vi "Serial Test.vi"() -> ()   [LabVIEW 2011]
uses:
  PID/Engine RPM/Engine RPM.lvclass
  PID/Throttle Position/Throttle Position.lvclass
  PID/Fuel Level Input/Fuel Level Input Folder/Fuel Level Input.lvclass
  PID/PID.lvclass
  PID/VIN/VIN Folder/VIN.lvclass
  <vilib>/Instr/_visa.llb/VISA Configure Serial Port (Instr).vi
panel:
  out "Fuel Level":dbl(knob) scale=0.0..100.0
  in  "Get All":bool
  out "Response":string
  out "Throttle":dbl(knob) scale=0.0..100.0
  out "Waveform Chart 2":cluster{"Result":dbl, "Result":dbl}(graph)
  out "RPM":dbl(knob) scale=0.0..5000.0
  out "Discard?":bool
  in  "milliseconds to wait":u32=250
  in  "VIN":bool
  in  "Polling":bool
  in  "Check All":bool
  out "number":u32
  in  "29-Bit CAN":bool[](array[boolean])
  in  "Send Button":bool
  in  "Command":string
  in  "Multicolumn Listbox 2":i32(listbox)=-1
  out "String":string="0100\r\r41 00 BE 7F A8 13 \r0120\r\r41 20 80 07 B0 11 \r0140\r\r41 40 FE D0 0C 00 \r0100\r41 00 BE 7F A8 13 \r0102\rNO DATA\r0103\r41 03 02 00 \r0104\r41 04 30 \r0105\r41 05 80 \r0106\r41 06 86 \r0109\rNO DATA\r010A\r41 0A 7D \r010B\r41 0B 22 \r010C\r41 0C 0A 1F \r010D\r41 0D 00 \r010E\r41 0E 8A \r010F\r41 0F 3D \r0110\r41 10 01 45 \r0112\rNO DATA\r0114\rNO DATA\r011B\rNO DATA\r011E\rNO DATA\r011F\r41 1F 03 A4 \r0120\r41 20 80 07 B0 11 \r012D\rNO DATA\r012E\r41 2E FF \r012F\r41 2F ED \r0130\r41 30 FF \r0132\rNO DATA\r0133\r41 33 65 \r013B\rNO DATA\r013F\rNO DATA\r0140\r41 40 FE D0 0C 00 \r0141\r41 41 00 07 E5 A5 \r0142\r41 42 37 FF \r0143\r41 43 00 29 \r0144\r41 44 7C AC \r0145\r41 45 04 \r0146\r41 46 31 \r0148\rNO DATA\r0149\r41 49 12 \r014B\rNO DATA\r0154\rNO DATA\r0155\r41 55 82 \r010C\r41 0C 0A 30 \r0111\r41 11 21 \r010C\r41 0C 0A 37 \r0111\r41 11 21 \r010C\r41 0C 0A 44 \r0111\r41 11 21 \r010C\r41 0C 0A 28 \r0111\r41 11 21 \r010C\r41 0C 0A 1B \r0111\r41 11 21 \r010C\r41 0C 0A 26 \r0111\r41 11 21 \r010C\r41 0C 0A 10 \r0111\r41 11 21 \r010C\r41 0C 0A 1B \r0111\r41 11 21 \r010C\r41 0C 0A 26 \r0111\r41 11 21 \r010C\r41 0C 0A 4F \r0111\r41 11 21 \r010C\r41 0C 0A 49 \r0111\r41 11 21 \r010C\r41 0C 0A 40 \r0111\r41 11 21 \r010C\r41 0C 0A 40 \r0111\r41 11 21 \r010C\r41 0C 0A 19 \r0111\r41 11 21 \r010C\r41 0C 0A 27 \r0111\r41 11 21 \r010C\r41 0C 0A 13 \r0111\r41 11 21 \r010C\r41 0C 09 FF \r0111\r41 11 21 \r010C\r41 0C 0A 20 \r0111\r41 11 21 \r010C\r41 0C 0A 50 \r0111\r41 11 21 \r010C\r41 0C 0A 38 \r0111\r41 11 21 \r010C\r41 0C 0A 18 \r0111\r41 11 21 \r010C\r41 0C 0A 0D \r0111\r41 11 21 \r010C\r41 0C 0A 26 \r0111\r41 11 21 \r010C\r41 0C 0A 30 \r0111\r41 11 21 \r010C\r41 0C 0A 29 \r0111\r41 11 21 \r010C\r41 0C 0A 31 \r0111\r41 11 21 \r010C\r41 0C 0A 24 \r0111\r41 11 21 \r010C\r41 0C 0A 26 \r0111\r41 11 21 \r010C\r41 0C 0A 23 \r0111\r41 11 21 \r010C\r41 0C 0A 25 \r0111\r41 11 21 \r010C\r41 0C 0A 14 \r0111\r41 11 21 \r010C\r41 0C 0A 39 \r0111\r41 11 21 \r010C\r41 0C 0A 0D \r0111\r41 11 21 \r010C\r41 0C 0A 00 \r0111\r41 11 21 \r010C\r41 0C 0A 29 \r0111\r41 11 21 \r010C\r41 0C 0A 25 \r0111\r41 11 21 \r010C\r41 0C 0A 22 \r0111\r41 11 21 \r010C\r41 0C 0A 2D \r0111\r41 11 21 \r010C\r41 0C 0A 40 \r0111\r41 11 21 \r010C\r41 0C 0A 44 \r0111\r41 11 21 \r010C\r41 0C 0A 30 \r0111\r41 11 21 \r010C\r41 0C 0A 2D \r0111\r41 11 21 \r010C\r41 0C 0A 33 \r0111\r41 11 21 \r010C\r41 0C 0A 17 \r0111\r41 11 21 \r010C\r41 0C 0A 34 \r0111\r41 11 21 \r010C\r41 0C 0A 2B \r0111\r41 11 21 \r010C\r41 0C 0A 46 \r0111\r41 11 21 \r010C\r41 0C 0A 1C \r0111\r41 11 21 \r010C\r41 0C 0A 10 \r0111\r41 11 21 \r010C\r41 0C 0A 2F \r0111\r41 11 21 \r010C\r41 0C 09 FB \r0111\r41 11 21 \r010C\r41 0C 0A 1B \r0111\r41 11 21 \r010C\r41 0C 0A 27 \r0111\r41 11 21 \r010C\r41 0C 0A 32 \r0111\r41 11 21 \r010C\r41 0C 0A 3D \r0111\r41 11 21 \r010C\r41 0C 0A 35 \r0111\r41 11 21 \r010C\r41 0C 0A 2E \r0111\r41 11 21 \r010C\r41 0C 0A 34 \r0111\r41 11 21 \r010C\r41 0C 0A 1E \r0111\r41 11 21 \r010C\r41 0C 0A 05 \r0111\r41 11 21 \r010C\r41 0C 0A 16 \r0111\r41 11 21 \r010C\r41 0C 0A 3B \r0111\r41 11 21 \r010C\r41 0C 0A 38 \r0111\r41 11 21 \r010C\r41 0C 0A 46 \r0111\r41 11 21 \r010C\r41 0C 0A 29 \r0111\r41 11 21 \r010C\r41 0C 0A 2F \r0111\r41 11 21 \r010C\r41 0C 0A 2C \r0111\r41 11 21 \r010C\r41 0C 0A 1D \r0111\r41 11 21 \r010C\r41 0C 0A 01 \r0111\r41 11 21 \r010C\r41 0C 0A 19 \r0111\r41 11 21 \r010C\r41 0C 0A 18 \r0111\r41 11 21 \r010C\r41 0C 0A 0F \r0111\r41 11 21 \r010C\r41 0C 0A 32 \r0111\r41 11 21 \r010C\r41 0C 0A 49 \r0111\r41 11 21 \r010C\r41 0C 0A 49 \r0111\r41 11 21 \r010C\r41 0C 0A 5A \r0111\r41 11 21 \r010C\r41 0C 0A 4F \r0111\r41 11 21 \r010C\r41 0C 0A 3C \r0111\r41 11 21 \r010C\r41 0C 0A 2A \r0111\r41 11 21 \r010C\r41 0C 0A 28 \r0111\r41 11 21 \r010C\r41 0C 0A 04 \r0111\r41 11 21 \r010C\r41 0C 0A 1B \r0111\r41 11 21 \r010C\r41 0C 0A 24 \r0111\r41 11 21 \r010C\r41 0C 0A 4B \r0111\r41 11 21 \r010C\r41 0C 0A 30 \r0111\r41 11 21 \r010C\r41 0C 0A 11 \r0111\r41 11 21 \r010C\r41 0C 0A 05 \r0111\r41 11 21 \r010C\r41 0C 0A 0C \r0111\r41 11 21 \r010C\r41 0C 0A 1E \r0111\r41 11 21 \r010C\r41 0C 0A 26 \r0111\r41 11 21 \r010C\r41 0C 0A 30 \r0111\r41 11 21 \r010C\r41 0C 0A 41 \r0111\r41 11 21 \r010C\r41 0C 0A 2C \r0111\r41 11 21 \r010C\r41 0C 0A 3B \r0111\r41 11 21 \r010C\r41 0C 0A 2F \r0111\r41 11 21 \r010C\r41 0C 0A 34 \r0111\r41 11 21 \r010C\r41 0C 0A 48 \r0111\r41 11 21 \r010C\r41 0C 0A 2B \r0111\r41 11 21 \r010C\r41 0C 0A 27 \r0111\r41 11 21 \r010C\r41 0C 0A 25 \r0111\r41 11 21 \r010C\r41 0C 0A 19 \r0111\r41 11 21 \r010C\r41 0C 0A 2C \r0111\r41 11 21 \r010C\r41 0C 0A 30 \r0111\r41 11 21 \r010C\r41 0C 0A 11 \r0111\r41 11 21 \r010C\r41 0C 0A 38 \r0111\r41 11 21 \r010C\r41 0C 0A 20 \r0111\r41 11 21 \r010C\r41 0C 0A 25 \r0111\r41 11 21 \r010C\r41 0C 0A 1C \r0111\r41 11 21 \r010C\r41 0C 0A 2B \r0111\r41 11 21 \r010C\r41 0C 0A 2E \r0111\r41 11 21 \r010C\r41 0C 0A 40 \r0111\r41 11 21 \r010C\r41 0C 0A 1A \r0111\r41 11 21 \r010C\r41 0C 0A 1F \r0111\r41 11 21 \r010C\r41 0C 0A 2F \r0111\r41 11 21 \r010C\r41 0C 0A 22 \r0111\r41 11 21 \r010C\r41 0C 0A 3C \r0111\r41 11 21 \r010C\r41 0C 0A 27 \r0111\r41 11 21 \r010C\r41 0C 0A 27 \r0111\r41 11 21 \r010C\r41 0C 0A 12 \r0111\r41 11 21 \r010C\r41 0C 0A 37 \r0111\r41 11 21 \r010C\r41 0C 0A 1E \r0111\r41 11 21 \r010C\r41 0C 0A 13 \r0111\r41 11 21 \r010C\r41 0C 0A 1C \r0111\r41 11 22 \r010C\r41 0C 0A 16 \r0111\r41 11 22 \r010C\r41 0C 0A 00 \r0111\r41 11 22 \r010C\r41 0C 0A 1B \r0111\r41 11 22 \r0902\r\r014 \r0902\r\r014 \r0902\r\r014 \r0902\r\r014 \r0900\r\r49 00 55 40 00 00 \r0901\r\rNO DATA\r0902\r\r014 \r"
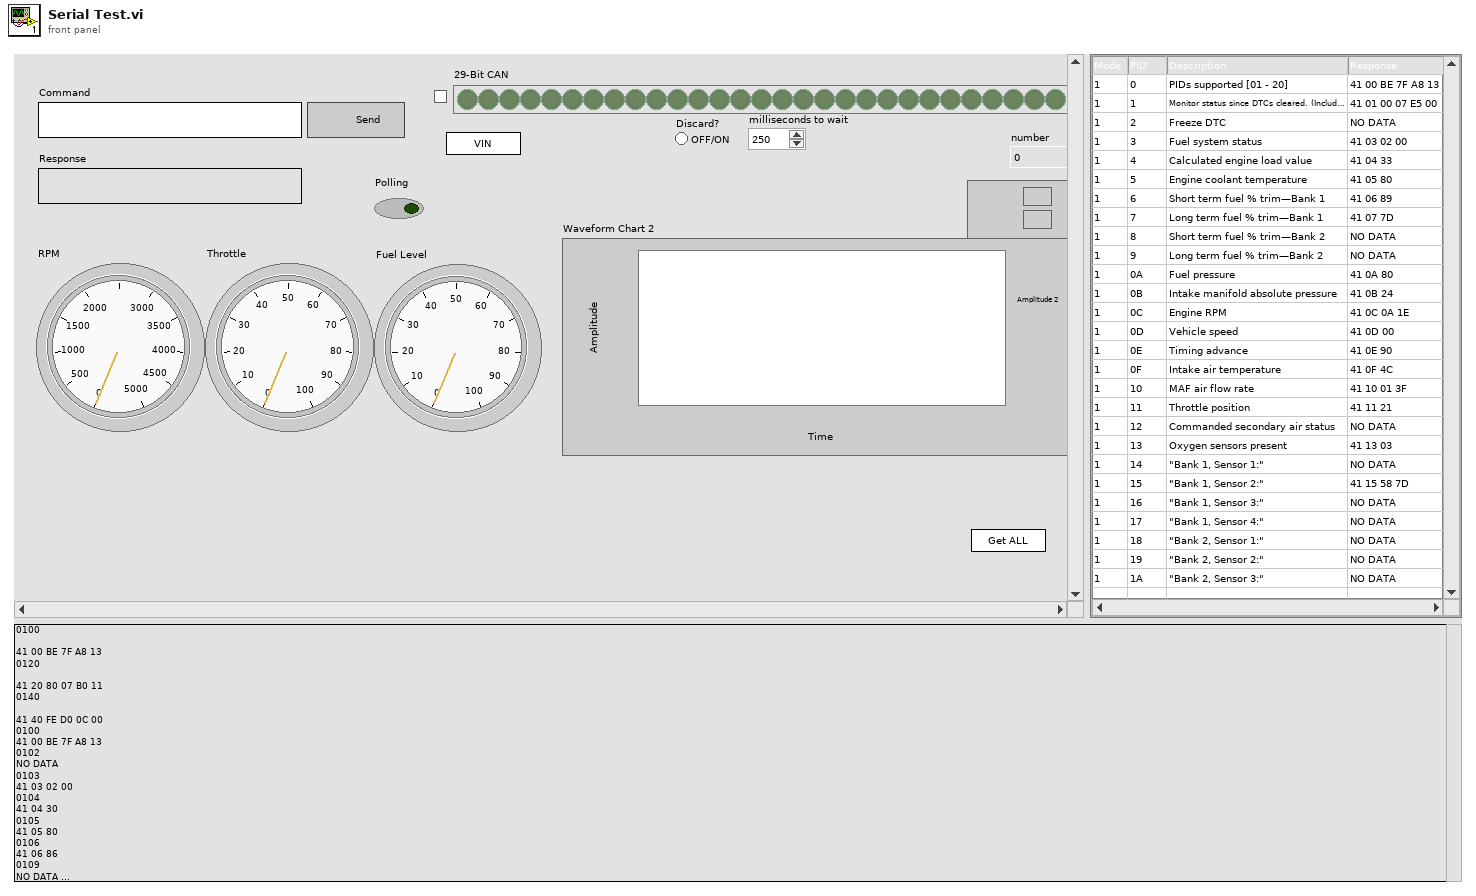
[diagram p1: front panel]
types:
  T1 = typedef "LVPoint32TypeDef.ctl" = cluster{"Horizontal":i32, "Vertical":i32}
  T2 = typedef "LVRowAndColumnTypeDef.ctl" = cluster{"Row":i32, "Column":i32}
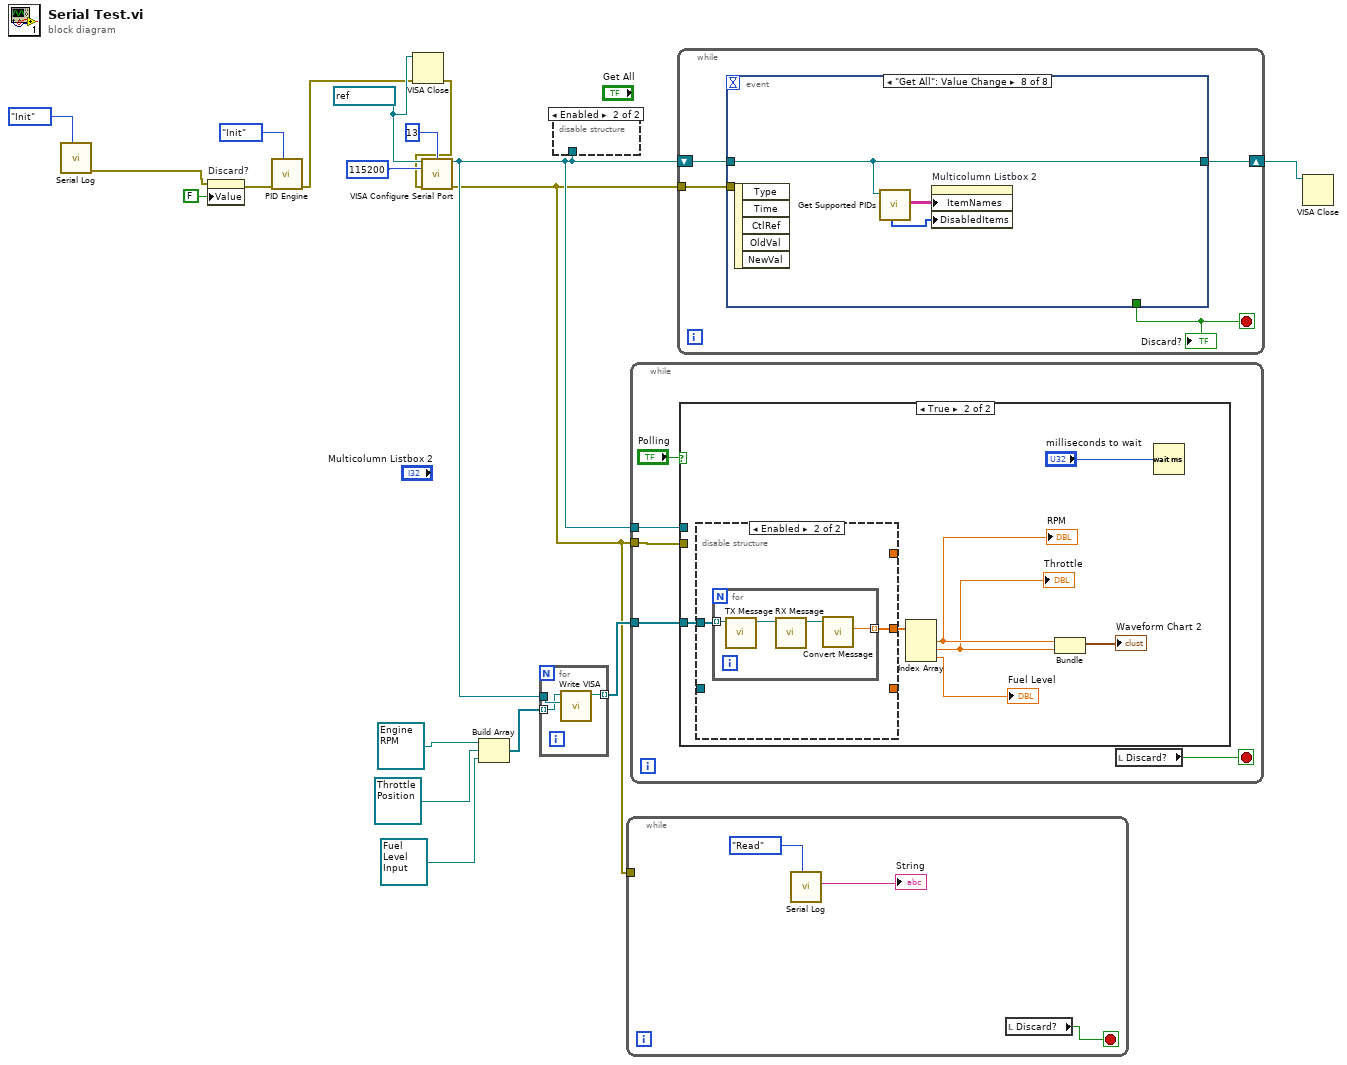
[diagram p0: block diagram]
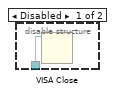
[diagram p2: hidden frame]
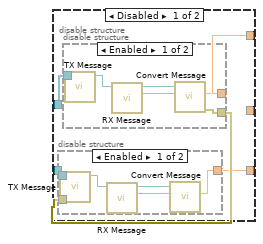
[diagram p4: hidden frame]
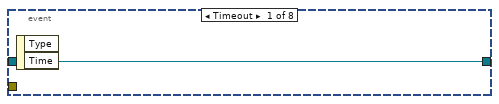
[diagram p7: hidden frame]
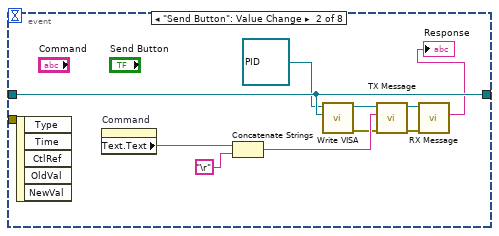
[diagram p8: hidden frame]
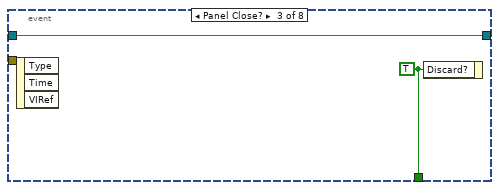
[diagram p9: hidden frame]
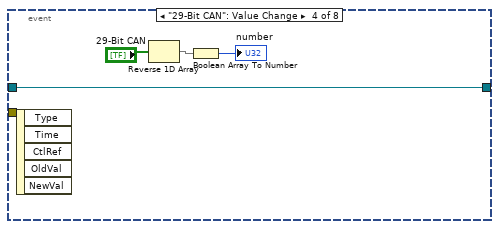
[diagram p10: hidden frame]
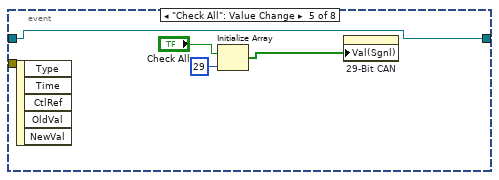
[diagram p11: hidden frame]
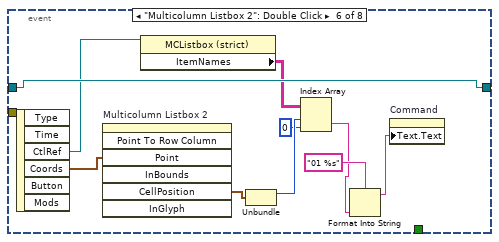
[diagram p12: hidden frame]
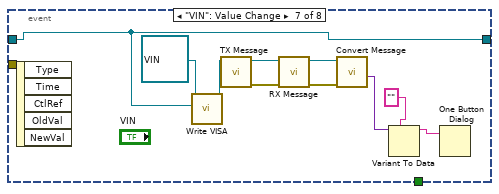
[diagram p13: hidden frame]
diagram:
  w4 = refnum<visa-resource-name> "COM3" ("VISA resource name")
  n1 = call "Serial Log.vi"("State"=enum16{"Init", "Write", "Read"}."Init") -> ("error out"=w6:errorcluster)  [unwired: 8 in, 2 out]
  n2 = property on="Discard?" class="Bool (strict)"(error in=w6, "Value"=FALSE ("Discard?")) -> (error out=w14:errorcluster)  [unwired: 1 in, 1 out]
  n3 = call "PID Engine.vi"("State"=enum16{"Init", "Get PID"}."Init", "error in (no error)"=w14) -> ("error out"=w2:errorcluster)  [unwired: 6 in, 3 out]
  n4 = VISA Close(VISA resource name=w4, error in (no error)=w2) -> (error out=w3:errorcluster)
  n5 = call-poly "VISA Configure Serial Port"("VISA resource name"=w4, "termination char\n(0xA = '\\n' = LF)"=u8 13 ("termination char\n(0xA = '\\n' = LF)"), "baud rate (9600)"=u32 115200, "error in (no error)"=w3) -> ("VISA resource name out"=w11:refnum<visa-resource-name>, "error out"=w7:errorcluster)  [unwired: 10 in]
  n6 = Build Array(refnum<class "Engine RPM.lvclass"> refnum ("Engine RPM.lvclass"), refnum<class "Throttle Position.lvclass"> refnum ("Throttle Position.lvclass"), refnum<class "Fuel Level Input.lvclass"> refnum ("Fuel Level Input.lvclass")) -> (w8:refnum<class "PID.lvclass">[])
  n7 = for {
    tunnel: [w21] -> w12 mode=indexing
    tunnel: w11 -> [w20]
    tunnel: w8 -> [w19] mode=indexing
    n8 = call "Write VISA.vi"("VISA"=w20, "PID in"=w19) -> ("PID out"=w21:refnum<class "PID.lvclass">)  [unwired: 8 in, 1 out]
  }
  n9 = disable-structure shown="Enabled" {
    disable-tunnel: w11 -> [w22 _]
    frame Disabled {
      n10 = VISA Close(VISA resource name=w22) -> ()  [unwired: 1 in, 1 out]
    }
    frame Enabled {
    }
  }
  n11 = while {
    tunnel: w7 -> [_]
    stop <- w25 stop-if-true
    n12 = call "Serial Log.vi"("State"=enum16{"Init", "Write", "Read"}."Read") -> ("Big String"=→"String":string)  [unwired: 8 in, 2 out]
    n13 = local read "Discard?"() -> (w25:bool)
  }
  n14 = while {
    tunnel: w11 -> [w30]
    tunnel: w7 -> [w29]
    tunnel: w12 -> [w26]
    stop <- w27 stop-if-true
    n15 = case shown="True" "Polling" {
      tunnel: w30 -> [_ _]
      tunnel: w29 -> [_ _]
      tunnel: w26 -> [_ w36]
      frame False {
      }
      frame True {
        n16 = disable-structure shown="Enabled" {
          disable-tunnel: w36 -> [w42 w56]
          disable-tunnel: _ -> [w41 _]
          disable-tunnel: [w39 _] -> _
          disable-tunnel: [w38 _] -> _
          disable-tunnel: [_ w55] -> w34
          frame Disabled {
            n17 = disable-structure shown="Enabled" {
              disable-tunnel: w42 -> [w48 _]
              disable-tunnel: [w44 _] -> w38
              disable-tunnel: [w43 _] -> w40
              frame Enabled {
                n18 = call-dynamic "TX Message.vi"("Engine RPM in"=w48) -> ("Engine RPM out"=w47:refnum<class "Engine RPM.lvclass">)  [unwired: 9 in, 1 out]
                n19 = call-dynamic "RX Message.vi"("PID in"=w47) -> ("String"=w45:string, "PID out"=w46:refnum<class "Engine RPM.lvclass">)  [unwired: 8 in, 1 out]
                n20 = call-dynamic "Convert Message.vi"(10:w45, "Engine RPM in"=w46) -> ("error out"=w43:errorcluster, "Result"=w44:dbl)  [unwired: 6 in, 2 out]
              }
              frame Disabled {
              }
            }
            n21 = disable-structure shown="Enabled" {
              disable-tunnel: w41 -> [w51 _]
              disable-tunnel: [w50 _] -> w39
              disable-tunnel: w40 -> [w49 _]
              frame Enabled {
                n22 = call-dynamic "TX Message.vi"("error in (no error)"=w49, "Throttle Position in"=w51) -> ("Throttle Position out"=w52:refnum<class "Throttle Position.lvclass">)  [unwired: 8 in, 1 out]
                n23 = call-dynamic "RX Message.vi"("PID in"=w52) -> ("String"=w54:string, "PID out"=w53:refnum<class "Throttle Position.lvclass">)  [unwired: 8 in, 1 out]
                n24 = call-dynamic "Convert Message.vi"(10:w54, "Throttle Position in"=w53) -> ("Result"=w50:dbl)  [unwired: 6 in, 3 out]
              }
              frame Disabled {
              }
            }
          }
          frame Enabled {
            n25 = for {
              tunnel: w56 -> [w58] mode=indexing
              tunnel: [w57] -> w55 mode=indexing
              n26 = call-dynamic "TX Message.vi"("PID in"=w58) -> ("PID out"=w59:refnum<class "PID.lvclass">)  [unwired: 9 in, 1 out]
              n27 = call-dynamic "RX Message.vi"("PID in"=w59) -> ("PID out"=w60:refnum<class "PID.lvclass">)  [unwired: 8 in, 2 out]
              n28 = call-dynamic "Convert Message.vi"("PID in"=w60) -> ("Result"=w57:dbl)  [unwired: 7 in, 3 out]
            }
          }
        }
        n29 = Index Array(array=w34) -> (element #1=w33:dbl, element #2=w32:dbl, element #3=→"Fuel Level":dbl)  [unwired: 3 in]
        "RPM" <- w33
        "Throttle" <- w32
        n30 = Bundle("Result"=w33, "Result"=w32) -> (→"Waveform Chart 2":cluster{"Result":dbl, "Result":dbl})  [unwired: 1 in]
        n31 = Wait (ms)(milliseconds to wait="milliseconds to wait") -> ()  [unwired: 1 out]
      }
    }
    n32 = local read "Discard?"() -> (w27:bool)
  }
  n33 = while {
    tunnel: w7 -> [w63]
    shift-right: [w61] -> w15
    shift-left: w11 -> [w64]
    stop <- w62 stop-if-true
    n34 = event shown="[7] \"Get All\": Value Change" {
      selector: _ -> [_ _ _ _ _ _ _ _]
      dyn-events: _ -> [_ _ _ _ _ _ _ _]
      timeout: _ -> [_ _ _ _ _ _ _ _]
      tunnel: w64 -> [w65 w72 w76 w78 w82 w95 w99 w107]
      tunnel: w63 -> [_ _ _ _ _ _ _ _]
      tunnel: [_ _ w77 _ _ _ _ _] -> w62
      tunnel: [w65 w72 w76 w78 w82 w95 w99 w107] -> w61
      event Timeout {
        n35 = event-data() -> ()  [unwired: 1 in, 2 out]
      }
      event "Send Button": Value Change {
        n36 = event-data() -> ()  [unwired: 1 in, 5 out]
        n37 = property on="Command" class="Str"() -> ("Text.Text"=w71:string)  [unwired: 2 in, 2 out]
        n38 = Concatenate Strings(w71, "\r") -> (w69:string)
        n39 = call "Write VISA.vi"("VISA"=w72, "PID in"=refnum<class "PID.lvclass"> refnum ("PID.lvclass")) -> ("error out"=w67:errorcluster, "PID out"=w73:refnum<class "PID.lvclass">)  [unwired: 8 in]
        n40 = call-dynamic "TX Message.vi"("error in (no error)"=w67, "variant"=w69, "PID in"=w73) -> ("error out"=w66:errorcluster, "PID out"=w74:refnum<class "PID.lvclass">)  [unwired: 7 in]
        n41 = call-dynamic "RX Message.vi"("error in (no error)"=w66, "PID in"=w74) -> ("String"=→"Response":string)  [unwired: 7 in, 2 out]
      }
      event Panel Close? {
        w77 = TRUE ("Discard?")
        n42 = event-data() -> ()  [unwired: 1 in, 3 out]
        n43 = event-data("Discard?"=w77) -> ()  [unwired: 1 in, 1 out]
      }
      event "29-Bit CAN": Value Change {
        n44 = event-data() -> ()  [unwired: 1 in, 5 out]
        n45 = Reverse 1D Array(array="29-Bit CAN") -> (reversed array=w79:bool[])
        n46 = Boolean Array To Number(Boolean array=w79) -> (number=→"number":u32)
      }
      event "Check All": Value Change {
        n47 = event-data() -> ()  [unwired: 1 in, 5 out]
        n48 = Initialize Array("Check All", 29 ("dimension size")) -> (w83:bool[])
        n49 = property on="29-Bit CAN" class="Arr (strict)"("Val(Sgnl)"=w83) -> ()  [unwired: 2 in, 2 out]
      }
      event "Multicolumn Listbox 2": Double Click {
        n50 = event-data() -> ("CtlRef"=w94:refnum<vi>, "Coords"=w86:T1)  [unwired: 1 in, 4 out]
        n51 = invoke on="Multicolumn Listbox 2" class="MCListbox (strict)" method="Point To Row Column"("Point"=w86) -> ("CellPosition"=w87:T2)  [unwired: 6 in, 6 out]
        n52 = property class="MCListbox (strict)"(reference=w94) -> ("ItemNames"=w93:string[][])  [unwired: 1 in, 2 out]
        n53 = Unbundle(w87) -> ("Row"=w92:i32)  [unwired: 1 out]
        n54 = Index Array(array=w93, index (row)=w92, index (col)=0 ("disabled index (col)")) -> (element=w89:string)
        n55 = Format Into String(format string="01 %s", w89) -> (resulting string=w88:string)  [unwired: 2 in, 1 out]
        n56 = property on="Command" class="Str"("Text.Text"=w88) -> ()  [unwired: 2 in, 2 out]
      }
      event "VIN": Value Change {
        n57 = event-data() -> ()  [unwired: 1 in, 5 out]
        n58 = call "Write VISA.vi"("VISA"=w99, "PID in"=refnum<class "VIN.lvclass"> refnum ("VIN.lvclass")) -> ("PID out"=w100:refnum<class "VIN.lvclass">)  [unwired: 8 in, 1 out]
        n59 = call-dynamic "TX Message.vi"("Engine RPM in"=w100) -> ("error out"=w102:errorcluster, "Engine RPM out"=w105:refnum<class "VIN.lvclass">)  [unwired: 9 in]
        n60 = call-dynamic "RX Message.vi"("error in (no error)"=w102, "VIN in"=w105) -> ("error out"=w103:errorcluster, "VIN out"=w104:refnum<class "VIN.lvclass">)  [unwired: 7 in, 1 out]
        n61 = call-dynamic "Convert Message.vi"("error in (no error)"=w103, "Engine RPM in"=w104) -> ("variant"=w98:variant)  [unwired: 6 in, 3 out]
        n62 = Variant To Data(type="", Variant=w98) -> (data=w96:string)  [unwired: 1 in, 1 out]
        n63 = One Button Dialog(message=w96) -> ()  [unwired: 1 in, 1 out]
      }
      event "Get All": Value Change {
        n64 = event-data() -> ()  [unwired: 1 in, 5 out]
        n65 = call "Get Supported PIDs.vi"("VISA"=w107) -> ("transposed array"=w108:string[][], "Disables"=w106:i32[])  [unwired: 7 in, 2 out]
        n66 = property on="Multicolumn Listbox 2" class="MCListbox (strict)"("ItemNames"=w108, "DisabledItems"=w106) -> ()  [unwired: 2 in, 2 out]
      }
    }
    "Discard?" <- w62
  }
  n67 = VISA Close(VISA resource name=w15) -> ()  [unwired: 1 in, 1 out]
